vi "dfd_nMAC_Dummy Core.vi"(0 "x":fxp<+/-,16,16>, 1 "reset":bool, 9 "input valid":bool) -> (4 "y":fxp<+/-,16,16>, 10 "output valid":bool, 14 "ready for input":bool)   [LabVIEW 2017]
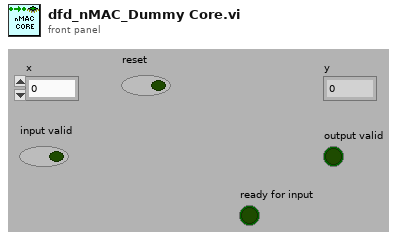
[diagram p1: front panel]
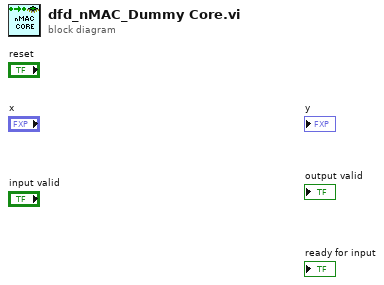
[diagram p0: block diagram]
diagram:
